vi "Robot_Enabled.vi"() -> (3 "Robot Enabled":bool)   [LabVIEW 2019]
uses:
  Robot Global Data.vi
  <vilib>/Rock Robotics/WPI/DriverStation/WPI_DriverStationRobotMode2.ctl
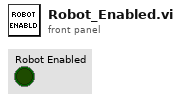
[diagram p1: front panel]
types:
  T1 = typedef "WPI_DriverStationRobotMode2.ctl" = enum16{"Autonomous Disabled", "Autonomous Enabled", "Teleop Disabled", "Teleop Enabled", "Disconnected", "Finish", "Test Disabled", "Test Enabled", "Emergency Stopped"}
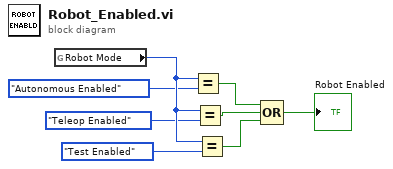
[diagram p0: block diagram]
diagram:
  n1 = global read "Robot Global Data.vi" "Robot Mode"() -> (w5:T1)
  n2 = Equal?(x=w5, y=WPI_DriverStationRobotMode2."Autonomous Enabled") -> (x = y?=w6:bool)
  n3 = Equal?(x=w5, y=WPI_DriverStationRobotMode2."Teleop Enabled") -> (x = y?=w7:bool)
  n4 = Equal?(x=w5, y=WPI_DriverStationRobotMode2."Test Enabled") -> (x = y?=w8:bool)
  n5 = Compound Arithmetic op=OR(w6, w7, w8) -> (→"Robot Enabled":bool)
